vi "runWaveFromFile.vi"() -> ()   [LabVIEW 2011, in "run.lvlib"]
uses:
  run.lvlib
  <vilib>/DAQmx/configure/trigger.llb/DAQmx Start Trigger (None).vi
  <vilib>/DAQmx/create/channels.llb/DAQmx Create Channel (AO-Voltage-Basic).vi
  <vilib>/DAQmx/configure/timing.llb/DAQmx Timing (Use Waveform).vi
  <vilib>/DAQmx/write.llb/DAQmx Write (Analog 1D DBL 1Chan NSamp).vi
  Channels/Digital/DigitalOutput.lvclass
panel:
  out "output cluster":T1 {"TimeStamps ms" format="%#_8g"}
  out "Samples":dbl
  out "min value":dbl
  out "Times ms":dbl[](array[numeric])
  in  "Stop":bool=TRUE
  out "Currents":dbl[](array[numeric])
  out "Delays":dbl[](array[numeric])
  in  "Current File":path=path "C:/Users/Administrator/Desktop/currentUpDown.txt"
  in  "Delay File":path=path "C:/Users/Administrator/Desktop/delays.txt"
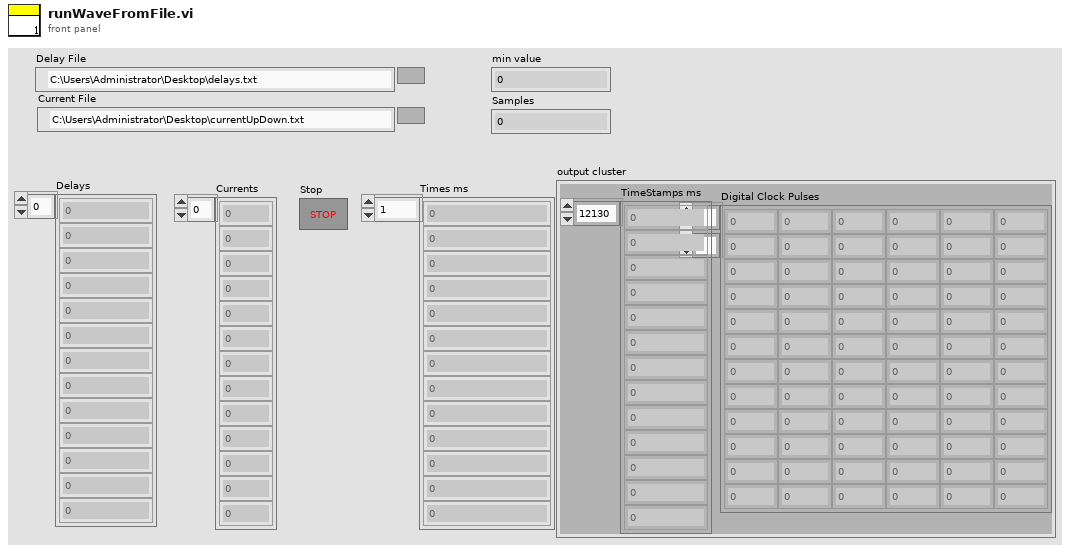
[diagram p1: front panel]
types:
  T1 = cluster{"TimeStamps ms":dbl[], "Digital Clock Pulses":i32[][]}
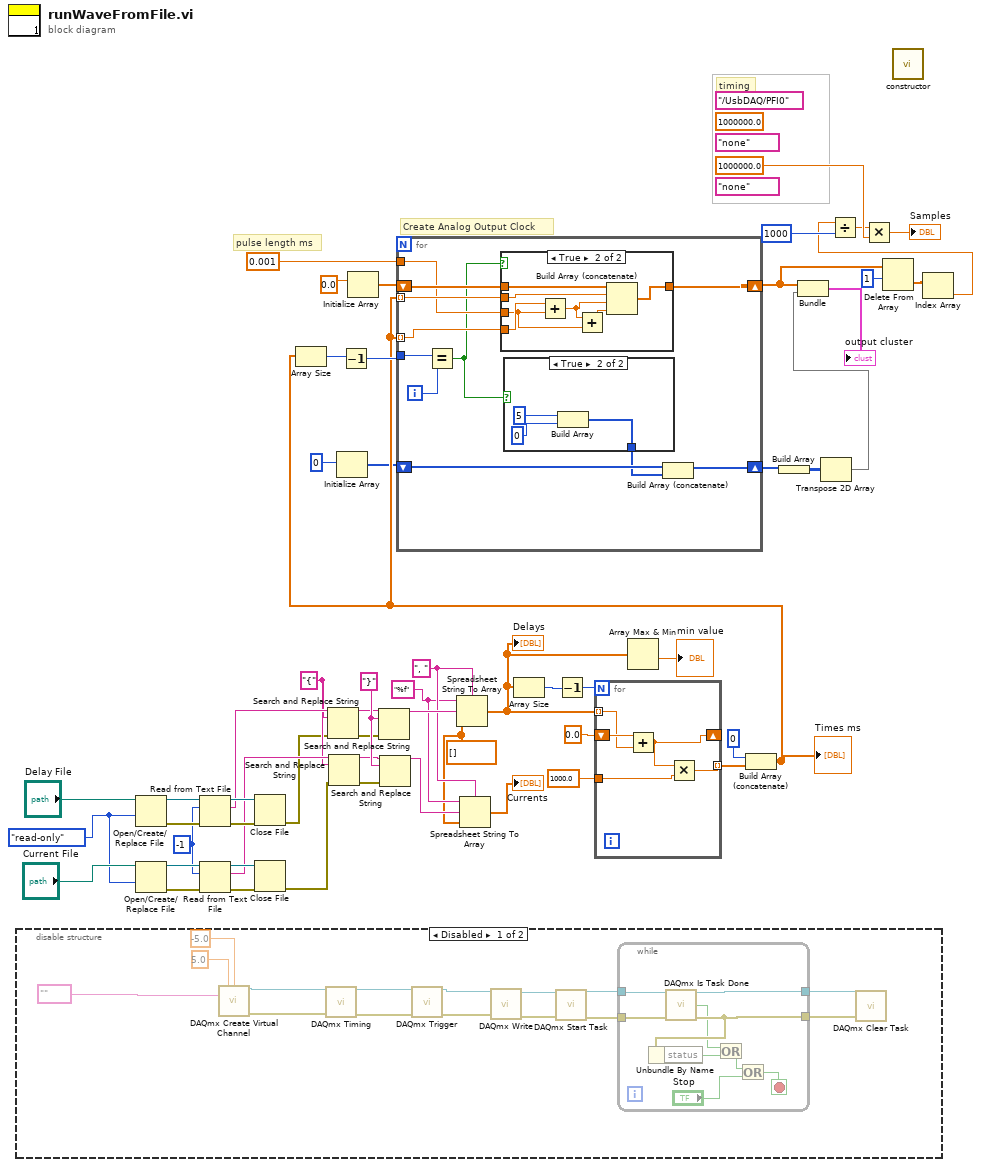
[diagram p0: block diagram]
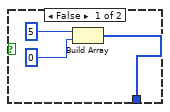
[diagram p2: hidden frame]
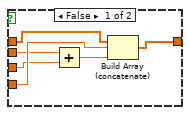
[diagram p3: hidden frame]
diagram:
  (unwired) "none" ("Stop trigger line")
  (unwired) "none" ("Start trigger line")
  (unwired) 1000000.0 ("Master Clock rate")
  (unwired) "/UsbDAQ/PFI0" ("Master Clock source")
  w30 = dbl[] [] ("array type (2D Dbl)")
  w32 = ", " ("delimiter (Tab)")
  w31 = "%f" ("format string")
  w41 = "}"
  w42 = "{"
  w46 = enum16{"read/write", "read-only", "write-only"}."read-only" ("access (0:read/write)")
  w45 = -1 ("count")
  # "timing"
  # "pulse length ms"
  # "Create Analog Output Clock"
  n1 = disable-structure shown="Disabled" {
    frame Disabled {
      n2 = call-poly <vilib>:"DAQmx Create Virtual Channel.vi"("maximum value"=5.0, "minimum value"=-5.0, "physical channels"=tag "") -> ("task out"=w66:refnum<k21>, "error out"=w65:errorcluster)  [unwired: 11 in]
      n3 = call-poly <vilib>:"DAQmx Timing.vi"("task/channels in"=w66, "error in"=w65) -> ("task out"=w67:refnum<k21>, "error out"=w64:errorcluster)  [unwired: 12 in]
      n4 = call-poly <vilib>:"DAQmx Trigger.vi"("task/channels in"=w67, "error in"=w64) -> ("task out"=w68:refnum<k21>, "error out"=w63:errorcluster)  [unwired: 12 in]
      n5 = call-poly <vilib>:"DAQmx Write.vi"("task/channels in"=w68, "error in"=w63) -> ("task out"=w69:refnum<k21>, "error out"=w62:errorcluster)  [unwired: 11 in, 1 out]
      n6 = call <vilib>:"DAQmx Start Task.vi"("task/channels in"=w69, "error in"=w62) -> ("task out"=w71:refnum<k21>, "error out"=w61:errorcluster)  [unwired: 12 in]
      n7 = while {
        tunnel: w71 -> [w79]
        tunnel: [w78] -> w70
        tunnel: w61 -> [w77]
        tunnel: [w76] -> w60
        stop <- w73 stop-if-true
        n8 = call <vilib>:"DAQmx Is Task Done.vi"("task/channels in"=w79, "error in"=w77) -> ("task out"=w78:refnum<k21>, "task done?"=w75:bool, "error out"=w76:errorcluster)  [unwired: 11 in]
        n9 = Unbundle By Name(w76) -> ("status"=w80:bool)
        n10 = Or(x=w75, y=w80) -> (x .or. y?=w74:bool)
        n11 = Or(x=w74, y="Stop") -> (x .or. y?=w73:bool)
      }
      n12 = call <vilib>:"DAQmx Clear Task.vi"("task in"=w70, "error in"=w60) -> ()  [unwired: 13 in, 1 out]
    }
    frame Enabled {
    }
  }
  n13 = Open/Create/Replace File(file path (use dialog)="Delay File", access (0:read/write)=w46) -> (refnum out=w56:refnum<file>, error out=w55:errorcluster)  [unwired: 4 in, 1 out]
  n14 = Open/Create/Replace File(file path (use dialog)="Current File", access (0:read/write)=w46) -> (refnum out=w51:refnum<file>, error out=w50:errorcluster)  [unwired: 4 in, 1 out]
  n15 = Read from Text File(file (use dialog)=w56, count=w45, error in=w55) -> (refnum out=w52:refnum<file>, text=w44:string, error out=w53:errorcluster)  [unwired: 1 in, 1 out]
  n16 = Read from Text File(file (use dialog)=w51, count=w45, error in=w50) -> (refnum out=w48:refnum<file>, text=w43:string, error out=w49:errorcluster)  [unwired: 1 in, 1 out]
  n17 = Close File(refnum=w52, error in=w53) -> (error out=w37:errorcluster)  [unwired: 1 out]
  n18 = Close File(refnum=w48, error in=w49) -> (error out=w36:errorcluster)  [unwired: 1 out]
  n19 = Search and Replace String(input string=w44, search string=w42, error in=w37) -> (result string=w40:string, error out=w38:errorcluster)  [unwired: 5 in, 2 out]
  n20 = Search and Replace String(input string=w43, search string=w42, error in=w36) -> (result string=w39:string, error out=w35:errorcluster)  [unwired: 5 in, 2 out]
  n21 = Initialize Array(0) -> (w12:i32[])  [unwired: 1 in]
  n22 = Initialize Array(0.0) -> (w20:dbl[])  [unwired: 1 in]
  n23 = Search and Replace String(input string=w40, search string=w41, error in=w38) -> (result string=w34:string)  [unwired: 5 in, 3 out]
  n24 = Search and Replace String(input string=w39, search string=w41, error in=w35) -> (result string=w33:string)  [unwired: 5 in, 3 out]
  n25 = Spreadsheet String To Array(delimiter (Tab)=w32, format string=w31, spreadsheet string=w34, array type (2D Dbl)=w30) -> (array=w23:dbl[])
  "Delays" <- w23
  n26 = Spreadsheet String To Array(delimiter (Tab)=w32, format string=w31, spreadsheet string=w33, array type (2D Dbl)=w30) -> (array=→"Currents":dbl[])
  n27 = Array Size(array=w23) -> (size(s)=w28:i32)
  n28 = Decrement(x=w28) -> (x-1=w27:i32)
  n29 = for {
    N: w27 -> [_]
    tunnel: w23 -> [w84] mode=indexing
    shift-right: [w82] -> _
    shift-left: 0.0 -> [w85]
    tunnel: [w83] -> w25 mode=indexing
    tunnel: 1000.0 ("y") -> [w81]
    n30 = Add(x=w85, y=w84) -> (x+y=w82:dbl)
    n31 = Multiply(x=w82, y=w81) -> (x*y=w83:dbl)
  }
  n32 = Array Max & Min(array=w23) -> (min value=→"min value":dbl)  [unwired: 3 out]
  n33 = Build Array (concatenate)(0, w25) -> (w14:dbl[])
  "Times ms" <- w14
  n34 = Array Size(array=w14) -> (size(s)=w19:i32)
  n35 = Decrement(x=w19) -> (x-1=w18:i32)
  n36 = for {
    shift-right: [w87] -> w4
    shift-left: w12 -> [w88]
    tunnel: w14 -> [w96] mode=indexing
    shift-right: [w95] -> w17
    shift-left: w20 -> [w94]
    tunnel: w14 -> [w93] mode=indexing
    tunnel: w18 -> [w92]
    tunnel: 0.001 -> [w90]
    i -> [w91]
    n37 = Equal?(x=w92, y=w91) -> (x = y?=w89:bool)
    n38 = case shown="True" w89 {
      tunnel: w96 -> [w108 w112]
      tunnel: [w106 w114] -> w95
      tunnel: w94 -> [w105 w115]
      tunnel: w93 -> [w104 w113]
      tunnel: w90 -> [w103 w109]
      frame False {
        n39 = Add(x=w104, y=w103) -> (x+y=w107:dbl)
        n40 = Build Array (concatenate)(w105, w108, w107) -> (w106:dbl[])
      }
      frame True {
        n41 = Add(x=w112, y=w109) -> (x+y=w111:dbl)
        n42 = Add(x=w111, y=w109) -> (x+y=w110:dbl)
        n43 = Build Array (concatenate)(w115, w113, w111, w110) -> (w114:dbl[])
      }
    }
    n44 = case shown="True" w89 {
      tunnel: [w97 w100] -> w86
      frame False {
        n45 = Build Array(5, 0) -> (w97:i32[])
      }
      frame True {
        n46 = Build Array(5, 0) -> (w100:i32[])
      }
    }
    n47 = Build Array (concatenate)(w88, w86) -> (w87:i32[])
  }
  n48 = Build Array(w4) -> (w3:i32[][])
  n49 = Transpose 2D Array(2D array=w3) -> (transposed array=w2:i32[][])
  n50 = Bundle(w17, w2) -> (→"output cluster":cluster{dbl[], i32[][]})  [unwired: 1 in]
  n51 = Delete From Array(array=w17, length=1) -> (deleted portion=w15:dbl[])  [unwired: 1 in, 1 out]
  n52 = call "constructor.vi"() -> ()  [unwired: 10 in, 2 out]
  n53 = Index Array(array=w15) -> (element=w7:dbl)  [unwired: 1 in]
  n54 = Divide(x=w7, y=1000) -> (x/y=w9:dbl)
  n55 = Multiply(x=w9, y=1000000.0 ("Scan rate")) -> (x*y=→"Samples":dbl)
